vi "Teardown.vi"(11 "Base Event jettl in":refnum<class "Base Event jettl.lvclass">) -> (3 "Base Event jettl out":refnum<class "Base Event jettl.lvclass">)   [LabVIEW 2021, in "jettl.lvlib" / "Base Event jettl.lvlib" / "Base Event jettl.lvclass"]
uses:
  Base Event jettl.lvclass
  State/Teardown State/Teardown State.lvclass
  C:/git/jettl/src/jettl/Base Event jettl/State/State/State.lvclass
  Base Event jettl.lvclass/Base Event jettl.ctl
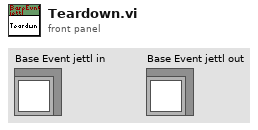
[diagram p1: front panel]
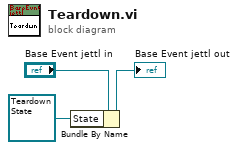
[diagram p0: block diagram]
diagram:
  n1 = Bundle By Name(cluster="Base Event jettl in", "State"=refnum<class "Teardown State.lvclass"> refnum ("jettl.lvlib:Teardown Event State.lvclass")) -> (→"Base Event jettl out":refnum<class "Base Event jettl.lvclass">)
